vi "Setup DecFrame Data.vi"(6 "Border Spacing":i16=-2, 7 "Monitor #":u16, 8 "Error":errorcluster, 9 "FPLocation":T1=enum."MID-CTR", 10 "Decoration Index":i32, 11 "(FP)":refnum<class "DecFrame_FP.lvclass">) -> (0 "Error Out":errorcluster, 3 "(FP) Out":refnum<class "DecFrame_FP.lvclass">)   [LabVIEW 2016, in "DecFrame_FP.lvclass"]
uses:
  DecFrame_FP.lvclass
  E:/~Data/FRC/Magic Trident/Code/UI LED Build file Interface/Utility/Universal Utility/FP/FPClass/(FP)/(FP).lvclass
  TypeDefs_Utility/ENUM RB_Pos_Quadrant Position.ctl
  DecFrame_FP.lvclass/DecFrame_FP.ctl
  (FP).lvclass
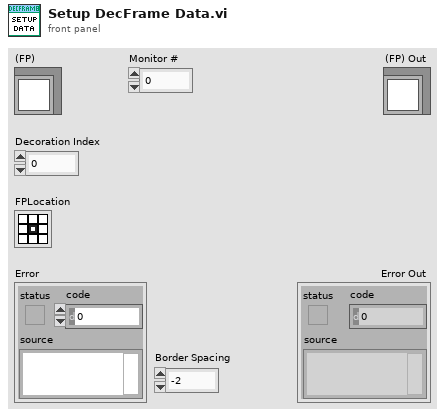
[diagram p1: front panel]
types:
  T1 = typedef "ENUM RB_Pos_Quadrant Position.ctl" = enum32{"LFT-TOP", "MID-TOP", "RGT-TOP", "LFT-CTR", "MID-CTR", "RGT-CTR", "LFT-BOT", "MID-BOT", "RGT-BOT"}
  T2 = typedef "LVRectTypeDef.ctl" = cluster{"Left":i16, "Top":i16, "Right":i16, "Bottom":i16}
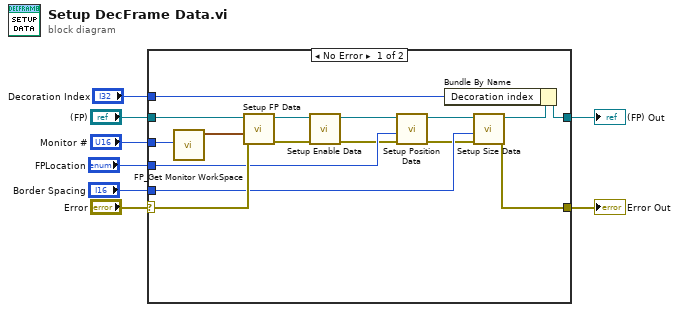
[diagram p0: block diagram]
diagram:
  n1 = case shown="No Error" "Error" {
    selector: "Error" -> [w23 w26]
    tunnel: [w9 w26] -> w7
    tunnel: [w15 w25] -> w5
    tunnel: "(FP)" -> [w24 w25]
    tunnel: "Monitor #" -> [w21 _]
    tunnel: "FPLocation" -> [w17 _]
    tunnel: "Decoration Index" -> [w14 _]
    tunnel: "Border Spacing" -> [w11 _]
    frame No Error {
      n2 = call "FP_Get Monitor WorkSpace.vi"("Monitor #"=w21) -> ("Disp.WkSpace Out"=w22:T2)  [unwired: 2 in]
      n3 = call "Setup FP Data.vi"("Error"=w23, "WkSpace"=w22, "(FP)"=w24) -> ("Error Out"=w20:errorcluster, "(FP) Out"=w19:refnum<class "DecFrame_FP.lvclass">)  [unwired: 7 in]
      n4 = call-dynamic "Setup Enable Data.vi"("Error"=w20, "(FP)"=w19) -> ("Error Out"=w16:errorcluster, "(FP) Out"=w18:refnum<class "DecFrame_FP.lvclass">)  [unwired: 8 in]
      n5 = call-dynamic "Setup Position Data.vi"("Error"=w16, "FPLocation"=w17, "(FP)"=w18) -> ("Error Out"=w10:errorcluster, "(FP) Out"=w13:refnum<class "DecFrame_FP.lvclass">)  [unwired: 7 in]
      n6 = call-dynamic "Setup Size Data.vi"("Error"=w10, "Border Spacing"=w11, "(FP)"=w13) -> ("Error Out"=w9:errorcluster, "(FP) Out"=w12:refnum<class "DecFrame_FP.lvclass">)  [unwired: 7 in]
      n7 = Bundle By Name(cluster=w12, "Decoration index"=w14) -> (w15:refnum<class "DecFrame_FP.lvclass">)
    }
    frame Error {
    }
  }
  "Error Out" <- w7
  "(FP) Out" <- w5
